vi "ber_qpsk.vi"() -> ()   [LabVIEW 2014]
uses:
  <vilib>/Analysis/NI_AALBase.lvlib
panel:
  out "Scatter plot":cluster{dbl[], dbl[]}(graph)
  out "SER":dbl
  out "BER":dbl
  in  "s3":dbl[](array[numeric])
  in  "s2":dbl[](array[numeric])
  in  "s1":dbl[](array[numeric])
  in  "s0":dbl[](array[numeric])
  in  "Number of bits":dbl
  in  "Eb/N0(dB)":dbl
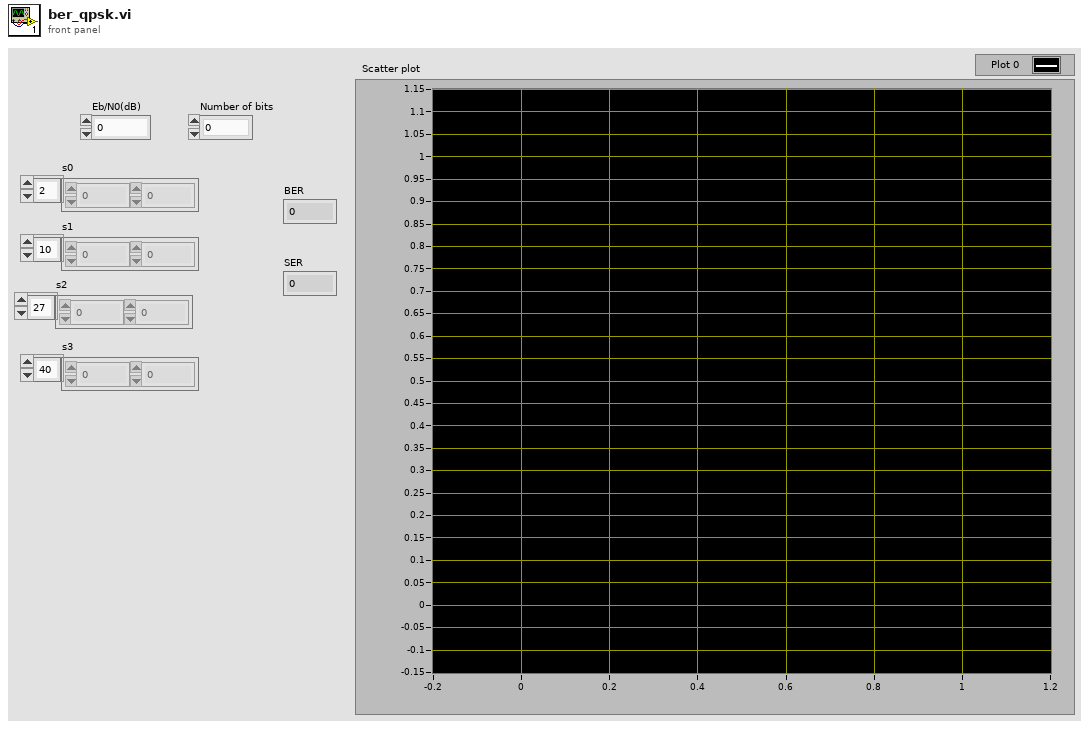
[diagram p1: front panel]
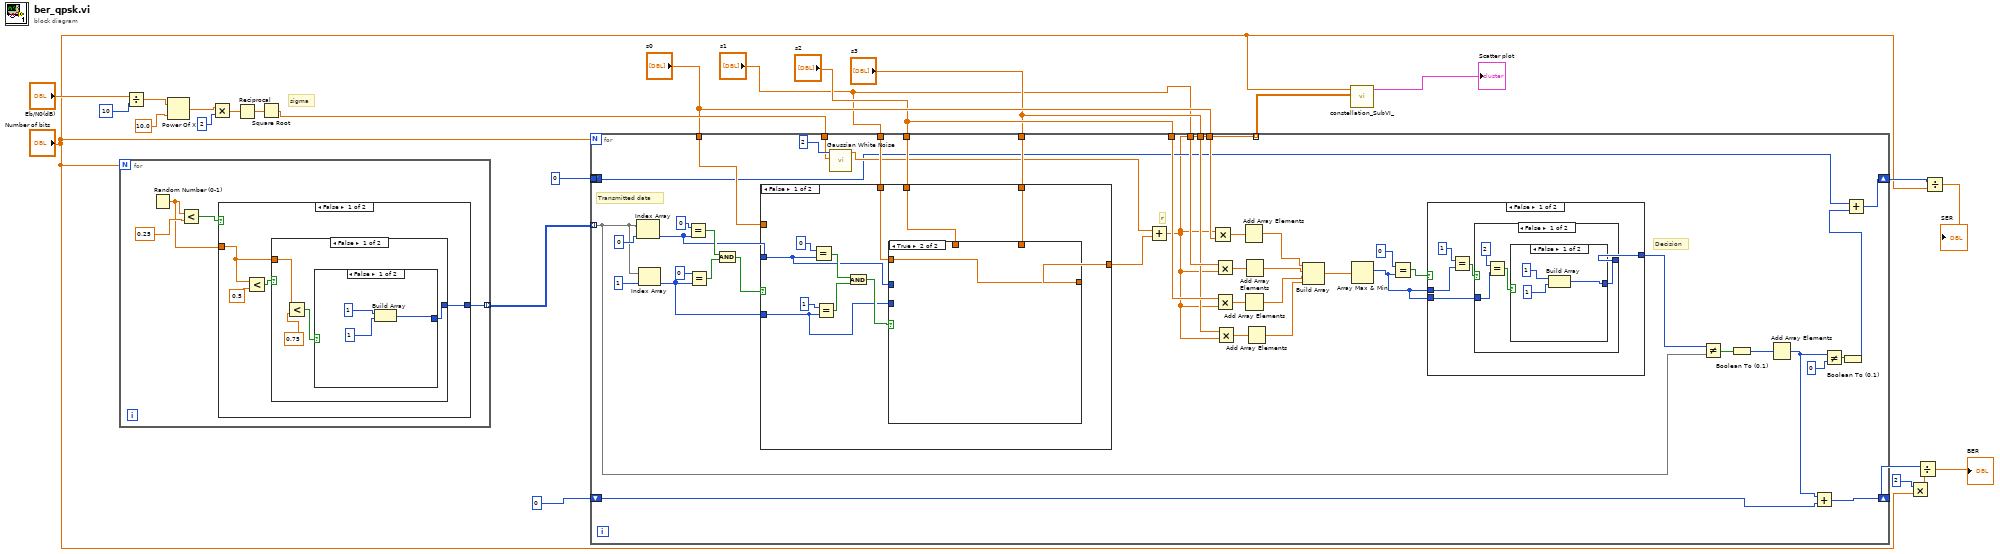
[diagram p0: block diagram]
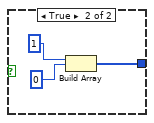
[diagram p2: hidden frame]
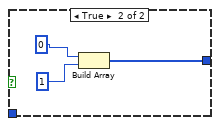
[diagram p3: hidden frame]
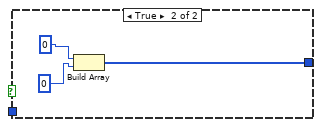
[diagram p4: hidden frame]
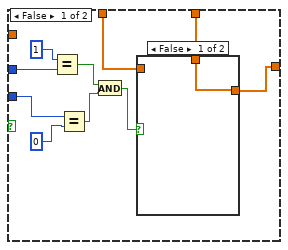
[diagram p5: hidden frame]
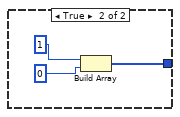
[diagram p8: hidden frame]
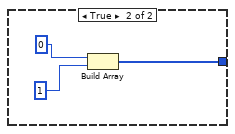
[diagram p9: hidden frame]
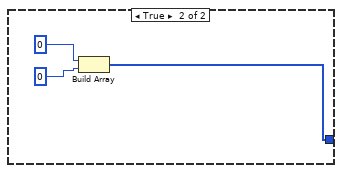
[diagram p10: hidden frame]
diagram:
  # "sigma"
  n1 = for {
    N: "Number of bits" -> [_]
    tunnel: [w26] -> w17 mode=indexing
    n2 = Random Number (0-1)() -> (number: 0 to 1=w27:dbl)
    n3 = Less?(x=w27, y=0.25) -> (x < y?=w29:bool)
    n4 = case shown="False" w29 {
      tunnel: w27 -> [w30 _]
      tunnel: [w31 w47] -> w26
      frame False {
        n5 = Less?(x=w30, y=0.5) -> (x < y?=w33:bool)
        n6 = case shown="False" w33 {
          tunnel: [w34 w44] -> w31
          tunnel: w30 -> [w37 _]
          frame False {
            n7 = Less?(x=w37, y=0.75) -> (x < y?=w35:bool)
            n8 = case shown="False" w35 {
              tunnel: [w38 w41] -> w34
              frame False {
                n9 = Build Array(1, 1) -> (w38:i32[])
              }
              frame True {
                n10 = Build Array(1, 0) -> (w41:i32[])
              }
            }
          }
          frame True {
            n11 = Build Array(0, 1) -> (w44:i32[])
          }
        }
      }
      frame True {
        n12 = Build Array(0, 0) -> (w47:i32[])
      }
    }
  }
  n13 = Divide(x="Eb/N0(dB)", y=10) -> (x/y=w23:dbl)
  n14 = Power Of X(1:10.0, 2:w23) -> (0:w22:dbl)
  n15 = Multiply(x=w22, y=2) -> (x*y=w20:dbl)
  n16 = Reciprocal(x=w20) -> (1/x=w19:dbl)
  n17 = Square Root(x=w19) -> (sqrt(x)=w18:dbl)
  n18 = for {
    N: "Number of bits" -> [_]
    tunnel: w18 -> [w94]
    tunnel: w17 -> [w62] mode=indexing
    tunnel: "s0" -> [w57]
    tunnel: "s1" -> [w84]
    tunnel: "s2" -> [w83]
    tunnel: "s3" -> [w82]
    tunnel: "s0" -> [w79]
    tunnel: "s1" -> [w78]
    tunnel: "s2" -> [w77]
    tunnel: "s3" -> [w76]
    shift-right: [w58] -> w12
    shift-left: 0 -> [w59]
    shift-right: [w51] -> w6
    shift-left: _ -> [w52]
    tunnel: 0 -> [_]
    tunnel: [w50] -> _ mode=indexing
    tunnel: [w50] -> w1 mode=indexing
    # "Transmitted data"
    # "Decision"
    # "r"
    n19 = Index Array(array=w62, index=0) -> (element=w86:i32)
    n20 = Index Array(array=w62, index=1) -> (element=w85:i32)
    n21 = Equal?(x=0, y=w86) -> (x = y?=w89:bool)
    n22 = Equal?(x=0, y=w85) -> (x = y?=w88:bool)
    n23 = And(x=w89, y=w88) -> (x .and. y?=w87:bool)
    n24 = case shown="False" w87 {
      tunnel: [w122 w141] -> w81
      tunnel: w57 -> [_ w141]
      tunnel: w86 -> [w120 _]
      tunnel: w85 -> [w119 _]
      tunnel: w84 -> [w121 _]
      tunnel: w83 -> [w118 _]
      tunnel: w82 -> [w117 _]
      frame False {
        n25 = Equal?(x=0, y=w120) -> (x = y?=w125:bool)
        n26 = Equal?(x=1, y=w119) -> (x = y?=w124:bool)
        n27 = And(x=w125, y=w124) -> (x .and. y?=w123:bool)
        n28 = case shown="True" w123 {
          tunnel: [w130 w140] -> w122
          tunnel: w121 -> [_ w140]
          tunnel: w120 -> [w136 _]
          tunnel: w119 -> [w134 _]
          tunnel: w118 -> [w129 _]
          tunnel: w117 -> [w128 _]
          frame False {
            n29 = Equal?(x=1, y=w136) -> (x = y?=w133:bool)
            n30 = Equal?(x=w134, y=0) -> (x = y?=w132:bool)
            n31 = And(x=w133, y=w132) -> (x .and. y?=w131:bool)
            n32 = case shown="False" w131 {
              tunnel: [w138 w139] -> w130
              tunnel: w129 -> [_ w139]
              tunnel: w128 -> [w138 _]
              frame False {
              }
              frame True {
              }
            }
          }
          frame True {
          }
        }
      }
      frame True {
      }
    }
    n33 = call <vilib>:"Gaussian White Noise.vi"("standard deviation"=w94, "samples"=2) -> ("Gaussian noise pattern"=w80:dbl[])  [unwired: 8 in, 1 out]
    n34 = Add(x=w80, y=w81) -> (x+y=w50:dbl[])
    n35 = Multiply(x=w50, y=w79) -> (x*y=w75:dbl[])
    n36 = Multiply(x=w78, y=w50) -> (x*y=w74:dbl[])
    n37 = Multiply(x=w77, y=w50) -> (x*y=w73:dbl[])
    n38 = Multiply(x=w76, y=w50) -> (x*y=w72:dbl[])
    n39 = Add Array Elements(numeric array=w75) -> (sum=w71:dbl)
    n40 = Add Array Elements(numeric array=w73) -> (sum=w69:dbl)
    n41 = Add Array Elements(numeric array=w74) -> (sum=w70:dbl)
    n42 = Add Array Elements(numeric array=w72) -> (sum=w68:dbl)
    n43 = Build Array(w71, w70, w69, w68) -> (w67:dbl[])
    n44 = Array Max & Min(array=w67) -> (max index (indices)=w64:i32)  [unwired: 3 out]
    n45 = Equal?(x=0, y=w64) -> (x = y?=w66:bool)
    n46 = case shown="False" w66 {
      tunnel: [w98 w114] -> w63
      tunnel: w64 -> [w99 _]
      tunnel: w64 -> [w96 _]
      frame False {
        n47 = Equal?(x=1, y=w99) -> (x = y?=w97:bool)
        n48 = case shown="False" w97 {
          tunnel: [w101 w111] -> w98
          tunnel: w96 -> [w103 _]
          frame False {
            n49 = Equal?(x=2, y=w103) -> (x = y?=w102:bool)
            n50 = case shown="False" w102 {
              tunnel: [w105 w108] -> w101
              frame False {
                n51 = Build Array(1, 1) -> (w105:i32[])
              }
              frame True {
                n52 = Build Array(1, 0) -> (w108:i32[])
              }
            }
          }
          frame True {
            n53 = Build Array(0, 1) -> (w111:i32[])
          }
        }
      }
      frame True {
        n54 = Build Array(0, 0) -> (w114:i32[])
      }
    }
    n55 = Not Equal?(x=w63, y=w62) -> (x != y?=w61:bool[])
    n56 = Boolean To (0,1)(Boolean=w61) -> (0, 1=w60:i16[])
    n57 = Add Array Elements(numeric array=w60) -> (sum=w56:i16)
    n58 = Add(x=w56, y=w59) -> (x+y=w58:i32)
    n59 = Not Equal?(x=w56, y=0) -> (x != y?=w54:bool)
    n60 = Boolean To (0,1)(Boolean=w54) -> (0, 1=w53:i16)
    n61 = Add(x=w52, y=w53) -> (x+y=w51:i16)
  }
  n62 = call "constellation_SubVI_.vi"("Array"=w1, "N"="Number of bits") -> ("Cluster"=→"Scatter plot":cluster{dbl[], dbl[]})  [unwired: 9 in]
  n63 = Multiply(x=2, y="Number of bits") -> (x*y=w10:dbl)
  n64 = Divide(x=w12, y=w10) -> (x/y=→"BER":dbl)
  n65 = Divide(x=w6, y="Number of bits") -> (x/y=→"SER":dbl)
